vi "p2.vi"() -> ()   [LabVIEW 2023, in "d23.lvlib"]
uses:
  d23.lvlib
  <vilib>/Utility/miscctls.llb/LVMapReplaceAction.ctl
  AOC/AOC.lvlib
panel:
  in  "Example":string="#.#####################\n#.......#########...###\n#######.#########.#.###\n###.....#.>.>.###.#.###\n###v#####.#v#.###.#.###\n###.>...#.#.#.....#...#\n###v###.#.#.#########.#\n###...#.#.#.......#...#\n#####.#.#.#######.#.###\n#.....#.#.#.......#...#\n#.#####.#.#.#########v#\n#.#...#...#...###...>.#\n#.#.#v#######v###.###v#\n#...#.>.#...>.>.#.###.#\n#####v#.#.###v#.#.###.#\n#.....#...#...#.#.#...#\n#.#########.###.#.#.###\n#...###...#...#...#.###\n###.###.#.###v#####v###\n#...#...#.#.>.>.#.>.###\n#.###.###.#.###.#.#v###\n#.....###...###...#...#\n#####################.#"
  in  "Example":bool=TRUE
  out "Answer":u64
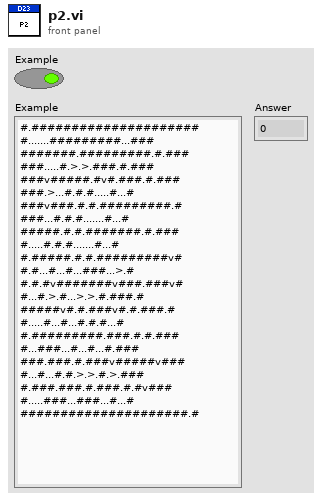
[diagram p1: front panel]
types:
  T1 = map{cluster{i32, i32}, cluster{"Slope":cluster{"x":i16, "y":i16}, "Directions":cluster{"x":i16, "y":i16}[], "Next Nodes":cluster{"RIGHT":cluster{"x":i16, "y":i16}, u64}[]}}
  T2 = cluster{"RIGHT":cluster{"x":i16, "y":i16}, u64}[]
  T3 = cluster{"RIGHT":cluster{"x":i16, "y":i16}, "UDLR (Vectors)":cluster{"x":i16, "y":i16}[], "Next Nodes":cluster{"RIGHT":cluster{"x":i16, "y":i16}, u64}[]}
  T4 = cluster{"Slope":cluster{"x":i16, "y":i16}, "Directions":cluster{"x":i16, "y":i16}[], "Next Nodes":cluster{"RIGHT":cluster{"x":i16, "y":i16}, u64}[]}
  T5 = cluster{"Location":cluster{i32, i32}, "Node Distance":u64, "Direction":cluster{"x":i16, "y":i16}}
  T6 = typedef "LVMapReplaceAction.ctl" = enum32{"Modify Entry only if found", "Add or Modify Entry", "Delete Entry"}
  T7 = cluster{"Location":cluster{i32, i32}, "Node Distance":u64}
  T8 = cluster{"Location":cluster{"x":i32, "y":i32}, "Node Distance":u64}[]
  T9 = cluster{cluster{i32, i32}, cluster{i32, i32}[], "Distance":u64}
  T10 = cluster{"RIGHT":cluster{"x":i16, "y":i16}, cluster{"x":i32, "y":i32}[], u64}
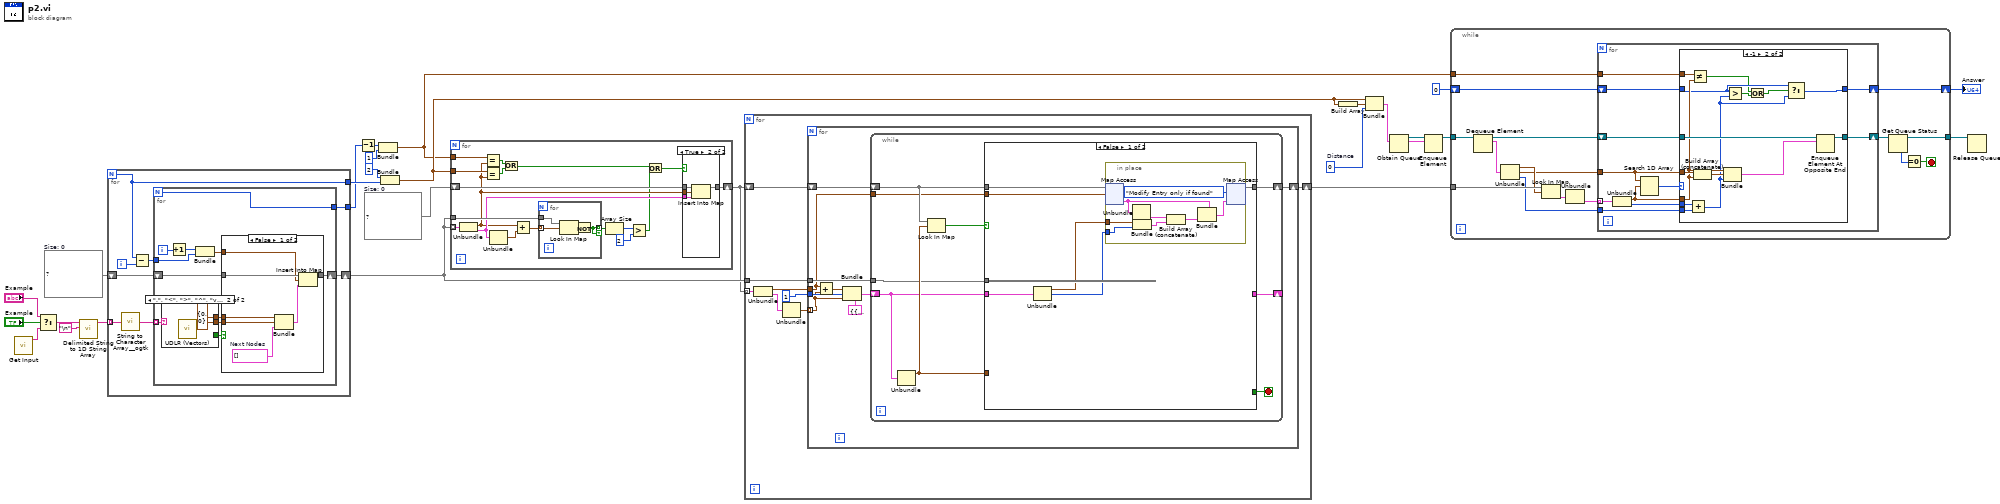
[diagram p0: block diagram]
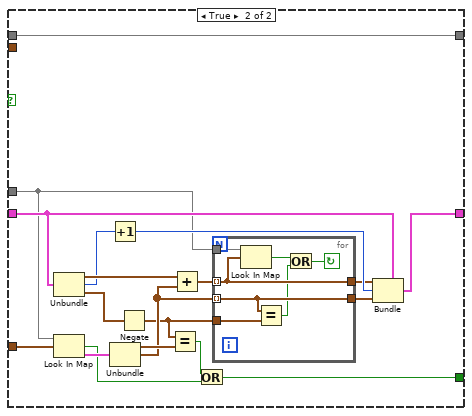
[diagram p3: hidden frame]
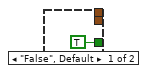
[diagram p5: hidden frame]
diagram:
  w8 = u64 0  # Distance
  w13 = T1 {}  # Size: 0
  w20 = T1 {}  # Size: 0
  n1 = call "Get Input.vi"() -> ("Input"=w26:string)  [unwired: 11 in]
  n2 = Select(t="Example", s="Example", f=w26) -> (s? t:f=w25:string)
  n3 = call <vilib>:"Delimited String to 1D String Array.vi"("delimiter"="\n", "delimited string"=w25) -> ("string array"=w21:string[])  [unwired: 9 in]
  n4 = for {
    N -> [w28]
    tunnel: w21 -> [w34] mode=indexing
    shift-right: [w29] -> w14
    shift-left: w20 -> [w30]
    tunnel: [w28] -> w18
    tunnel: [w27] -> w17
    i -> [w32]
    n5 = call <userlib>:"String to Character Array__ogtk.vi"("Input String"=w34) -> ("Character Array"=w33:string[])
    n6 = Subtract(x=w28, y=w32) -> (x-y=w31:i32)
    n7 = for {
      N -> [w35]
      tunnel: w33 -> [w37] mode=indexing
      tunnel: w31 -> [w43]
      shift-right: [w42] -> w29
      shift-left: w30 -> [w41]
      tunnel: [w35] -> w27
      i -> [w45]
      n8 = case shown="\".\", \"<\", \">\", \"^\", \"v\"" w37 {
        tunnel: [_ w48] -> w39
        tunnel: [TRUE _] -> w38
        tunnel: [_ cluster{"x":i16, "y":i16} {"x"=0, "y"=0} ("RIGHT")] -> w36
        frame "False", Default {
        }
        frame ".", "<", ">", "^", "v" {
          n9 = call "UDLR (Vectors).vi"() -> ("UDLR (Vectors)"=w48:cluster{"x":i16, "y":i16}[])  [unwired: 11 in]
        }
      }
      n10 = Increment(x=w45) -> (x+1=w44:i32)
      n11 = Bundle(w44, w43) -> (w40:cluster{i32, i32})  [unwired: 1 in]
      n12 = case shown="False" w38 {
        tunnel: [w55 w56] -> w42
        tunnel: w41 -> [w54 w56]
        tunnel: w40 -> [w53 _]
        tunnel: w39 -> [w52 _]
        tunnel: w36 -> [w49 _]
        frame False {
          w50 = T2 []  # Next Nodes
          n13 = Bundle("RIGHT"=w49, "UDLR (Vectors)"=w52, "Next Nodes"=w50) -> (w51:T3)  [unwired: 1 in]
          n14 = Insert Into Map(map in=w54, key=w53, value=w51) -> (map out=w55:T1)  [unwired: 2 out]
        }
        frame True {
        }
      }
    }
  }
  n15 = Decrement(x=w17) -> (x-1=w15:i32)
  n16 = Bundle(w15, 1) -> (w4:cluster{i32, i32})  [unwired: 1 in]
  n17 = Bundle(2, w18) -> (w6:cluster{i32, i32})  [unwired: 1 in]
  n18 = for {
    tunnel: w14 -> [w74] mode=indexing
    tunnel: w14 -> [w73]
    shift-right: [w66] -> w12
    shift-left: w13 -> [w67]
    tunnel: w4 -> [w64]
    tunnel: w6 -> [w63]
    n19 = Unbundle(w74) -> ("Location"=w62:cluster{i32, i32}, "Info"=w65:T4)
    n20 = Equal?(x=w64, y=w62) -> (x = y?=w60:bool)
    n21 = Equal?(x=w63, y=w62) -> (x = y?=w61:bool)
    n22 = Unbundle(w65) -> ("Directions"=w72:cluster{"x":i16, "y":i16}[])  [unwired: 2 out]
    n23 = Or(x=w60, y=w61) -> (x .or. y?=w59:bool)
    n24 = Add(x=w62, y=w72) -> (x+y=w71:cluster{i32, i32}[])
    n25 = for {
      tunnel: w71 -> [w82] mode=indexing
      tunnel: w73 -> [w83]
      tunnel: [w80] -> w70 mode=indexing if=w80
      n26 = Look In Map(map=w83, key=w82) -> (key not found?=w81:bool)  [unwired: 1 in, 1 out]
      n27 = Not(x=w81) -> (.not. x?=w80:bool)
    }
    n28 = Array Size(array=w70) -> (size(s)=w69:i32)
    n29 = Greater?(x=w69, y=2) -> (0:w58:bool)
    n30 = Or(x=w59, y=w58) -> (x .or. y?=w57:bool)
    n31 = case shown="True" w57 {
      tunnel: w67 -> [w75 w79]
      tunnel: [w75 w78] -> w66
      tunnel: w62 -> [_ w77]
      tunnel: w65 -> [_ w76]
      frame False {
      }
      frame True {
        n32 = Insert Into Map(map in=w79, key=w77, value=w76) -> (map out=w78:T1)  [unwired: 2 out]
      }
    }
  }
  n33 = for {
    tunnel: w14 -> [w91]
    shift-right: [w84] -> w11
    shift-left: w12 -> [w85]
    tunnel: w12 -> [w89] mode=indexing
    n34 = Unbundle(w89) -> ("Location"=w88:cluster{i32, i32}, "Info"=w87:T4)
    n35 = Unbundle(w87) -> ("Directions"=w86:cluster{"x":i16, "y":i16}[])  [unwired: 2 out]
    n36 = for {
      tunnel: u64 1 -> [w98]
      tunnel: w88 -> [w92]
      tunnel: w86 -> [w94] mode=indexing
      tunnel: w91 -> [w99]
      shift-right: [w95] -> w84
      shift-left: w85 -> [w96]
      n37 = Add(x=w92, y=w94) -> (x+y=w93:cluster{i32, i32})
      n38 = Bundle(cluster=T5 {"Location"={0, 0}, "Node Distance"=0, "Direction"={"x"=0, "y"=0}}, "Location"=w93, "Node Distance"=w98, "Direction"=w94) -> (w97:T5)
      n39 = while {
        shift-right: [w103] -> _
        shift-left: w97 -> [w106]
        tunnel: w99 -> [w108]
        tunnel: w92 -> [w102]
        shift-right: [w101] -> w95
        shift-left: w96 -> [w105]
        stop <- w104 stop-if-true
        n40 = Unbundle(w106) -> ("Location"=w109:cluster{i32, i32})  [unwired: 2 out]
        n41 = Look In Map(map=w105, key=w109) -> (key not found?=w107:bool)  [unwired: 1 in, 1 out]
        n42 = case shown="False" w107 {
          tunnel: w108 -> [_ w132]
          tunnel: [_ w137] -> w103
          tunnel: w109 -> [_ w140]
          tunnel: w106 -> [w114 w133]
          tunnel: w105 -> [w113 w131]
          tunnel: [_ w134] -> w104
          tunnel: [w112 w131] -> w101
          tunnel: w102 -> [w111 _]
          frame False {
            n43 = Unbundle(w114) -> ("Location"=w115:cluster{i32, i32}, "Node Distance"=w110:u64)  [unwired: 1 out]
            n44 = in-place {
              in-place-border: w115 -> [w118]
              in-place-border: w110 -> [w117]
              n45 = in-place-map #1(w113, w111) -> (w122:T4)  [unwired: 1 in, 1 out]
              n46 = Unbundle(w122) -> ("Next Nodes"=w123:T2)  [unwired: 2 out]
              n47 = Bundle("Location"=w118, "Node Distance"=w117) -> (w116:T7)  [unwired: 1 in]
              n48 = Build Array (concatenate)(w123, w116) -> (w121:T8)
              n49 = Bundle(cluster=w122, "Next Nodes"=w121) -> (w120:T4)  [unwired: 2 in]
              n50 = in-place-map #1(w120, LVMapReplaceAction."Modify Entry only if found" ("action")) -> (w112:T1)  [unwired: 2 out]
            }
          }
          frame True {
            n51 = Unbundle(w133) -> ("Location"=w125:cluster{i32, i32}, "Node Distance"=w124:u64, "Direction"=w139:cluster{"x":i16, "y":i16})
            n52 = Look In Map(map=w132, key=w140) -> (key not found?=w135:bool, value=w142:T4)  [unwired: 1 in]
            n53 = Increment(x=w124) -> (x+1=w138:u64)
            n54 = Unbundle(w142) -> ("Slope"=w141:cluster{"x":i16, "y":i16}, "Directions"=w128:cluster{"x":i16, "y":i16}[])  [unwired: 1 out]
            n55 = Negate(x=w139) -> (-x=w126:cluster{"x":i16, "y":i16})
            n56 = Equal?(x=w126, y=w141) -> (x = y?=w136:bool)
            n57 = Add(x=w125, y=w128) -> (x+y=w130:cluster{i32, i32}[])
            n58 = Or(x=w136, y=w135) -> (x .or. y?=w134:bool)
            n59 = for {
              tunnel: w132 -> [w149]
              tunnel: w130 -> [w148] mode=indexing
              tunnel: [w148] -> w129
              tunnel: w128 -> [w146] mode=indexing
              tunnel: [w146] -> w127
              tunnel: w126 -> [w145]
              stop <- w144 continue-if-true
              n60 = Look In Map(map=w149, key=w148) -> (key not found?=w147:bool)  [unwired: 1 in, 1 out]
              n61 = Equal?(x=w146, y=w145) -> (x = y?=w143:bool)
              n62 = Or(x=w147, y=w143) -> (x .or. y?=w144:bool)
            }
            n63 = Bundle(cluster=w133, "Location"=w129, "Node Distance"=w138, "Direction"=w127) -> (w137:T5)
          }
        }
      }
    }
  }
  n64 = Build Array(w6) -> (w5:cluster{i32, i32}[])
  n65 = Bundle(w6, w5, "Distance"=w8) -> (w9:T9)  [unwired: 1 in]
  n66 = Obtain Queue(element data type=w9) -> (queue out=w10:refnum<queue>)  [unwired: 4 in, 2 out]
  n67 = Enqueue Element(queue=w10, element=w9) -> (queue out=w7:refnum<queue>)  [unwired: 2 in, 2 out]
  n68 = while {
    tunnel: w11 -> [w165]
    tunnel: w7 -> [w164]
    tunnel: w4 -> [w153]
    tunnel: [w152] -> w3
    shift-right: [w150] -> w1
    shift-left: u64 0 ("x+y") -> [w151]
    stop <- w154 stop-if-true
    n69 = Dequeue Element(queue=w164) -> (queue out=w157:refnum<queue>, element=w163:T9)  [unwired: 2 in, 2 out]
    n70 = Unbundle(w163) -> (w162:cluster{i32, i32}, w159:cluster{i32, i32}[], "Distance"=w158:u64)
    n71 = Look In Map(map=w165, key=w162) -> (value=w161:T4)  [unwired: 1 in, 1 out]
    n72 = Unbundle(w161) -> ("Next Nodes"=w160:T2)  [unwired: 2 out]
    n73 = for {
      tunnel: w160 -> [w176] mode=indexing
      tunnel: w159 -> [w171]
      tunnel: w158 -> [w174]
      tunnel: w153 -> [w168]
      shift-right: [w169] -> w156
      shift-left: w157 -> [w172]
      shift-right: [w166] -> w150
      shift-left: w151 -> [w167]
      n74 = Unbundle(w176) -> ("RIGHT"=w170:cluster{"x":i16, "y":i16}, w173:u64)
      n75 = Search 1D Array(1D array=w171, element=w170) -> (index of element=w175:i32)  [unwired: 1 in]
      n76 = case shown="-1" w175 {
        tunnel: w174 -> [_ w189]
        tunnel: w173 -> [_ w190]
        tunnel: w172 -> [w178 w193]
        tunnel: w171 -> [_ w192]
        tunnel: w170 -> [_ w186]
        tunnel: [w178 w188] -> w169
        tunnel: w168 -> [_ w187]
        tunnel: w167 -> [w177 w184]
        tunnel: [w177 w182] -> w166
        frame Default {
        }
        frame -1 {
          n77 = Add(x=w190, y=w189) -> (x+y=w183:u64)
          n78 = Not Equal?(x=w187, y=w186) -> (x != y?=w180:bool)
          n79 = Build Array (concatenate)(w192, w186) -> (w191:cluster{"x":i32, "y":i32}[])
          n80 = Bundle("RIGHT"=w186, w191, w183) -> (w185:T10)  [unwired: 1 in]
          n81 = Greater?(x=w184, y=w183) -> (0:w181:bool)
          n82 = Or(x=w180, y=w181) -> (x .or. y?=w179:bool)
          n83 = Select(t=w184, s=w179, f=w183) -> (s? t:f=w182:u64)
          n84 = Enqueue Element At Opposite End(queue=w193, element=w185) -> (queue out=w188:refnum<queue>)  [unwired: 2 in, 2 out]
        }
      }
    }
    n85 = Get Queue Status(queue=w156) -> (queue out=w152:refnum<queue>, # elements in queue=w155:i32)  [unwired: 2 in, 6 out]
    n86 = Equal To 0?(x=w155) -> (x = 0?=w154:bool)
  }
  "Answer" <- w1
  n87 = Release Queue(queue=w3) -> ()  [unwired: 2 in, 3 out]
